vi "Close_Devices_Main_v2.vi"(8 "error in":errorcluster, 11 "Resources":T1 {"ZI ModHandle"."ModHandle" format="0x%08x"; "ZI ModHandle"."Conn" format="0x%08x"; "ZI Handle"."Handle" format="0x%08x"; "ZI Handle"."Conn" format="0x%08x"}) -> (0 "error out":errorcluster)   [LabVIEW 2021]
uses:
  Resources_v2.ctl
  <instrlib>/Zurich Instruments LabOne/Public/ziTypeHandle.ctl
  <instrlib>/Zurich Instruments LabOne/Public/Modules/ziTypeModHandle.ctl
  <instrlib>/Zurich Instruments LabOne/Zurich Instruments LabOne.lvlib
  <instrlib>/Keithley 622x LV 2009/Keithley 622x.lvlib
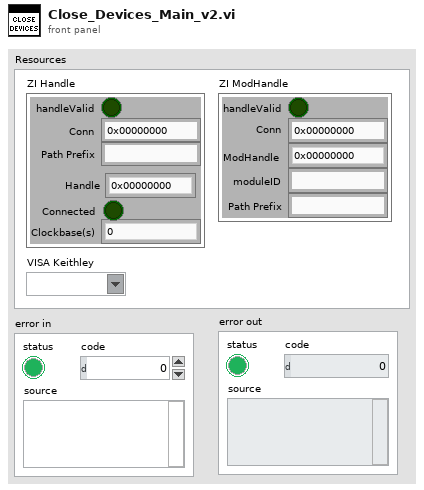
[diagram p1: front panel]
types:
  T1 = typedef "Resources_v2.ctl" = cluster{"ZI Handle":T2, "ZI ModHandle":T3, "VISA Keithley":refnum<visa-resource-name>}
  T2 = typedef "Zurich Instruments LabOne.lvlib/ziTypeHandle.ctl" = cluster{"handleValid":bool, "Conn":u64, "Path Prefix":string, "Handle":u64, "Clockbase(s)":dbl, "Connected":bool}
  T3 = typedef "Zurich Instruments LabOne.lvlib/ziTypeModHandle.ctl" = cluster{"handleValid":bool, "Conn":u64, "ModHandle":u64, "moduleID":string, "Path Prefix":string}
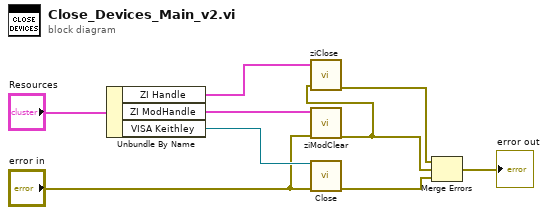
[diagram p0: block diagram]
diagram:
  n1 = Unbundle By Name("Resources") -> ("ZI Handle"=w7:T2, "ZI ModHandle"=w8:T3, "VISA Keithley"=w9:refnum<visa-resource-name>)
  n2 = call <instrlib>:"ziModClear.vi"("Error In"="error in", "ziModHandle In"=w8) -> ("Error Out"=w2:errorcluster)  [unwired: 7 in, 1 out]
  n3 = call <instrlib>:"ziClose.vi"("Error In"=w2, "Handle In"=w7) -> ("Error Out"=w5:errorcluster)  [unwired: 2 in, 1 out]
  n4 = call <instrlib>:"Close.vi"("VISA resource name"=w9, "error in (no error)"="error in") -> ("error out"=w4:errorcluster)  [unwired: 13 in]
  n5 = Merge Errors(w5, w2, w4) -> (→"error out":errorcluster)
